vi "PI_SPA.vi"(8 "Value":u16, 9 "Register":string, 10 "Axis":string, 11 "Commandset in":string[](array[string])) -> (3 "Commandset out":string[](array[string]))   [LabVIEW 8.6]
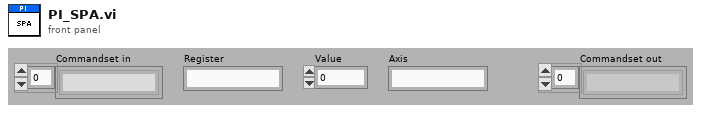
[diagram p1: front panel]
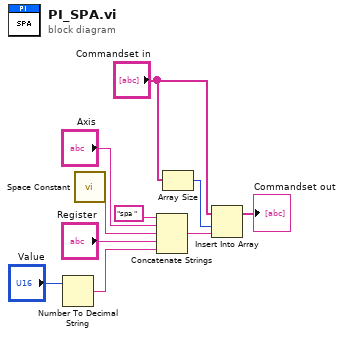
[diagram p0: block diagram]
diagram:
  n1 = Number To Decimal String(number="Value") -> (decimal integer string=w6:string)  [unwired: 1 out]
  n2 = call <vilib>:"Space Constant.vi"() -> ("String"=w4:string)
  n3 = Concatenate Strings("spa " ("new element/subarray"), "Axis", w4, "Register", w6) -> (w2:string)
  n4 = Array Size(array="Commandset in") -> (size(s)=w9:i32)
  n5 = Insert Into Array(array="Commandset in", index=w9, new element=w2) -> (→"Commandset out":string[])
